vi "ConfigAcquisition.vi"(8 "error in (no error)":errorcluster, 11 "NIScope in":refnum<class "NIScope.lvclass">) -> (0 "error out":errorcluster, 3 "NIScope out":refnum<class "NIScope.lvclass">)   [LabVIEW 2018, in "ScopePlugins.lvlib" / "NIScope.lvclass"]
uses:
  NIScope.lvclass
  Y:/Projects/PMUCal/Modules/Scope/ScopePlugins/ScopePluginBaseClass/ScopePluginsBase.lvclass
  ScopePluginBaseClass/ScopePluginsBase.lvclass/ScopePluginsBase.ctl
  ScopePluginBaseClass/Accessors/Read Connected.vi
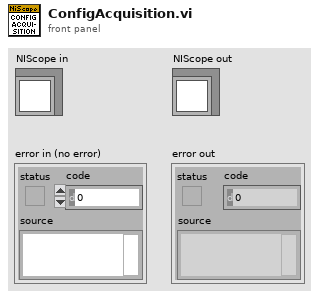
[diagram p1: front panel]
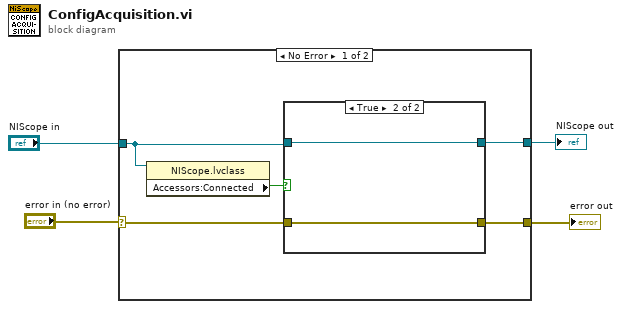
[diagram p0: block diagram]
diagram:
  n1 = case shown="No Error" "error in (no error)" {
    selector: "error in (no error)" -> [w8 w14]
    tunnel: "NIScope in" -> [w5 w15]
    tunnel: [w7 w14] -> w2
    tunnel: [w6 w15] -> w1
    frame No Error {
      n2 = property class="NIScope.lvclass"(reference=w5) -> ("Accessors:Connected"=w9:bool)  [unwired: 1 in, 2 out]
      n3 = case shown="True" w9 {
        tunnel: w8 -> [w11 w12]
        tunnel: [w11 w12] -> w7
        tunnel: [w10 w13] -> w6
        tunnel: w5 -> [w10 w13]
        frame False {
        }
        frame True {
        }
      }
    }
    frame Error {
    }
  }
  "error out" <- w2
  "NIScope out" <- w1
